vi "dotNET Constructor Map.vi"   [LabVIEW 2021]
uses:
  System.Core
panel:
  # "See block diagram"
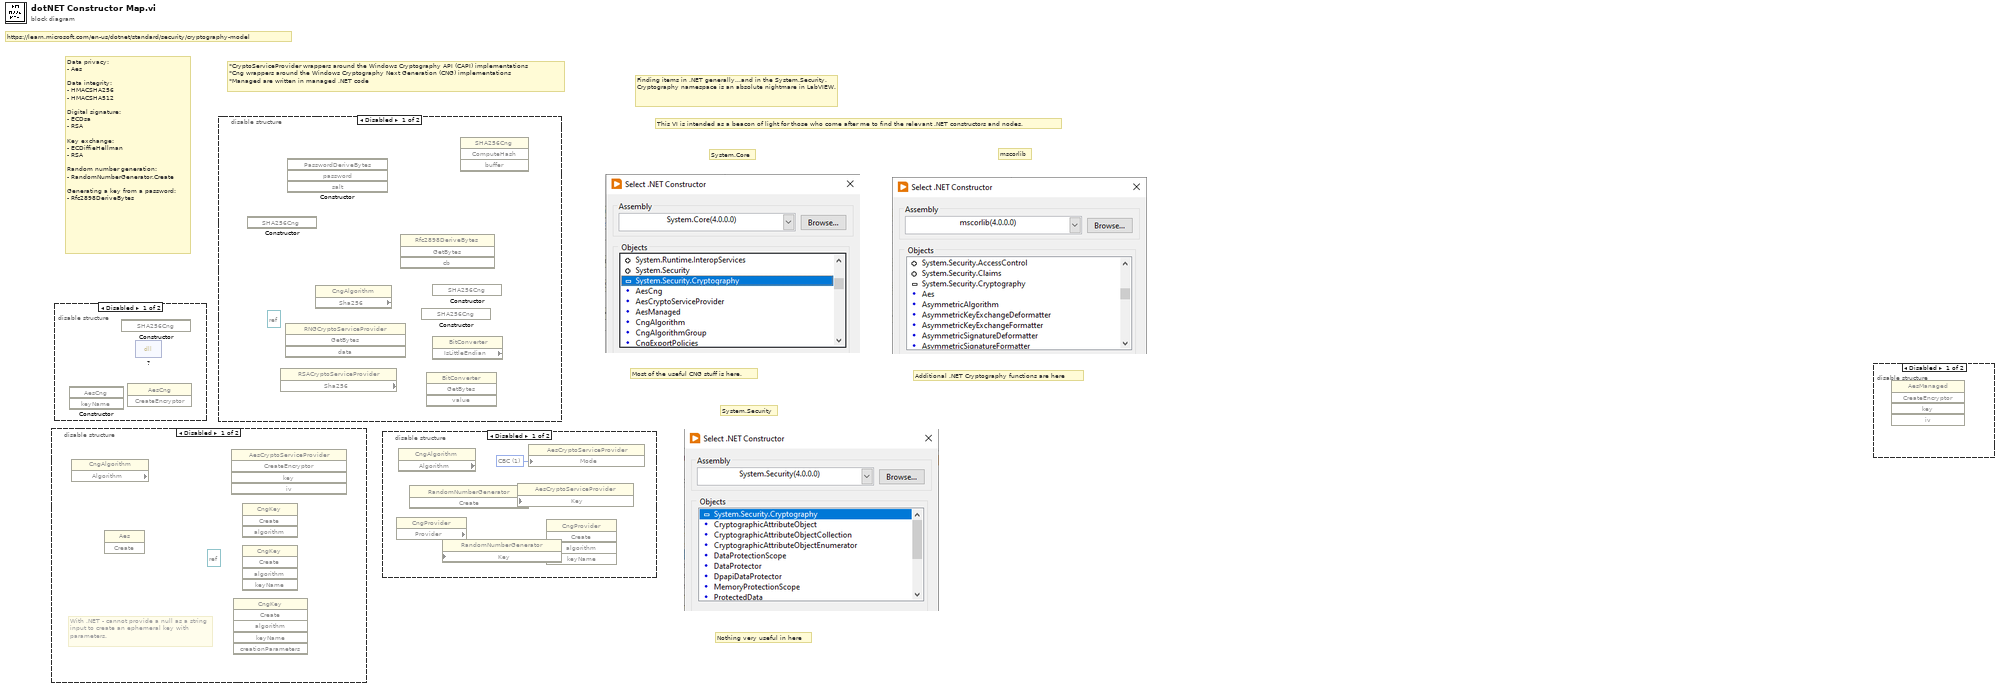
[diagram p0: block diagram]
diagram:
  # "*CryptoServiceProvider wrappers around the Windows Cryptography API (CAPI) implementations\n*Cng wrappers around the Windows Cryptography Next Generation (CNG) implementations\n*Managed are written in managed .NET code"
  # "Nothing very useful in here"
  # "Additional .NET Cryptography functions are here"
  # "Most of the useful CNG stuff is here."
  # "System.Security"
  # "mscorlib"
  # "System.Core"
  # "This VI is intended as a beacon of light for those who come after me to find the relevant .NET constructors and nodes."
  # "Finding items in .NET generally...and in the System.Security.Cryptography namespace is an absolute nightmare in LabVIEW."
  # "https://learn.microsoft.com/en-us/dotnet/standard/security/cryptography-model"
  # "Data privacy:\n- Aes\n\nData integrity:\n- HMACSHA256\n- HMACSHA512\n\nDigital signature:\n- ECDsa\n- RSA\n\nKey exchange:\n- ECDiffieHellman\n- RSA\n\nRandom number generation:\n- RandomNumberGenerator.Create\n\nGenerating a key from a password:\n- Rfc2898DeriveBytes"
  n1 = disable-structure shown="Disabled" {
    frame Disabled {
      (unwired) refnum<k24> refnum ("reference")
      # "With .NET - cannot provide a null as a string input to create an ephemeral key with parameters."
      n2 = property class="CngAlgorithm" props=["Algorithm"]() -> ()  [unwired: 2 in, 3 out]
      n3 = invoke class="Aes" method="Create"() -> ()  [unwired: 3 in, 3 out]
      n4 = invoke class="AesCryptoServiceProvider" method="CreateEncryptor"() -> ()  [unwired: 5 in, 5 out]
      n5 = invoke class="CngKey" method="Create"() -> ()  [unwired: 6 in, 6 out]
      n6 = invoke class="CngKey" method="Create"() -> ()  [unwired: 4 in, 4 out]
      n7 = invoke class="CngKey" method="Create"() -> ()  [unwired: 5 in, 5 out]
    }
    frame Enabled {
    }
  }
  n8 = disable-structure shown="Disabled" {
    frame Disabled {
      n9 = constructor class="AesCng"() -> ()  [unwired: 4 in, 4 out]
      n10 = constructor class="SHA256Cng"() -> ()  [unwired: 3 in, 3 out]
      n11 = invoke class="AesCng" method="CreateEncryptor"() -> ()  [unwired: 3 in, 3 out]
      n12 = dll-call lib="?" fn="?"() -> ()  [unwired: 4 in, 2 out]
    }
    frame Enabled {
    }
  }
  n13 = disable-structure shown="Disabled" {
    frame Disabled {
      (unwired) refnum<k24> refnum ("algorithm")
      n14 = constructor class="SHA256Cng"() -> ()  [unwired: 3 in, 3 out]
      n15 = property class="RSACryptoServiceProvider" props=["Sha256"]() -> ()  [unwired: 2 in, 3 out]
      n16 = invoke class="RNGCryptoServiceProvider" method="GetBytes"() -> ()  [unwired: 4 in, 4 out]
      n17 = constructor class="PasswordDeriveBytes"() -> ()  [unwired: 5 in, 5 out]
      n18 = property class="CngAlgorithm" props=["Sha256"]() -> ()  [unwired: 2 in, 3 out]
      n19 = invoke class="Rfc2898DeriveBytes" method="GetBytes"() -> ()  [unwired: 4 in, 4 out]
      n20 = constructor class="SHA256Cng"() -> ()  [unwired: 3 in, 3 out]
      n21 = invoke class="BitConverter" method="GetBytes"() -> ()  [unwired: 4 in, 4 out]
      n22 = constructor class="SHA256Cng"() -> ()  [unwired: 3 in, 3 out]
      n23 = property class="BitConverter" props=["IsLittleEndian"]() -> ()  [unwired: 2 in, 3 out]
      n24 = invoke class="SHA256Cng" method="ComputeHash"() -> ()  [unwired: 4 in, 4 out]
    }
    frame Enabled {
    }
  }
  n25 = disable-structure shown="Disabled" {
    frame Disabled {
      w1 = 1 items=["CBC"=1, "ECB"=2, "OFB"=3, "CFB"=4, "CTS"=5] ("Mode")
      n26 = property class="CngProvider" props=["Provider"]() -> ()  [unwired: 2 in, 3 out]
      n27 = property class="CngAlgorithm" props=["Algorithm"]() -> ()  [unwired: 2 in, 3 out]
      n28 = invoke class="RandomNumberGenerator" method="Create"() -> ()  [unwired: 3 in, 3 out]
      n29 = property class="RandomNumberGenerator" props=["Key"]() -> ()  [unwired: 3 in, 2 out]
      n30 = property class="AesCryptoServiceProvider" props=["Key"]() -> ()  [unwired: 3 in, 2 out]
      n31 = property class="AesCryptoServiceProvider"("Mode"=w1) -> ()  [unwired: 2 in, 2 out]
      n32 = invoke class="CngProvider" method="Create"() -> ()  [unwired: 5 in, 5 out]
    }
    frame Enabled {
    }
  }
  n33 = disable-structure shown="Disabled" {
    frame Disabled {
      n34 = invoke class="AesManaged" method="CreateEncryptor"() -> ()  [unwired: 5 in, 5 out]
    }
    frame Enabled {
    }
  }
